vi "excavator1D_singleSet.vi"(4 "x Max":dbl format="%#_13g", 6 "x Min":dbl format="%#_13g", 9 "Limits":bool=TRUE, 10 "Index Selection":dbl[](graph)=[-5.5039248036337095e-05, 0.002307601651409641, 0.0019375252973986789, 0.0020539827004540713, 0.0018766465480439364, 0.002005471562733874, 0.0019512440951075405, 0.0019016214297153055, 0.0020314427267294375, 0.0021225218602921813, 0.0020813973096664995, 0.0022190025250893087, 0.001999956712825224, 0.0021371180017013105, 0.0022027734317816793, 0.0022226846020203085, 0.0021817092376295475, 0.0022948075755266474, 0.0022634134918916972, 0.0024800556187983603, 0.0024709631223231556, 0.0024774496152531354, 0.0025178377341944723, 0.002528270776383579, 0.0024779048399068415, 0.0024436424602754412, 0.002515299420338124, 0.002657992171589285, 0.002703678625402972, 0.0027635940117761494, 0.0026640722469892355, 0.0028217502404004335, 0.002767086564563215, 0.0027189288404770194, 0.002773431036621332, 0.002864902134751901, 0.0028404979093465954, 0.0028498102794401346, 0.0029649439034983515, 0.002844457468017936, 0.0028746504918672144, 0.0026685349992476405, 0.002743897819891572, 0.0028248644433915616, 0.002763545874040574, 0.0026688438490964474, 0.0026700377056840807, 0.0024837456992827358, 0.002380804240237922, 0.0024809345486573875, 0.0024448799376841635, 0.002402537123998627, 0.0024637061171233652, 0.0022932857275009154, 0.002131347142858431, 0.0022557196440175175, 0.0021800588699989023, 0.0021162735123652966, 0.0020641911192797124, 0.00210531207267195, 0.0022086400946136563, 0.001933887047925964, 0.002116878272499889, 0.0022065737983211872, 0.0020789780362974854, 0.0020607836777344346, 0.002077205339446664, 0.0021651801478583367, 0.0022058752714656294, 0.0022308619110845028, 0.002125738380709663, 0.0022845100960694254, 0.0021997722215019166, 0.0022234479489270597, 0.002461879176553339, 0.0025202257151249797, 0.0027610767225269227, 0.0025679582846350967, 0.0027760936878621577, 0.0029153746319934724, 0.002828183607198298, 0.002911771065555513, 0.002850099717034027, 0.003011852188501507, 0.002978001633891836, 0.0030534794554114343, 0.0032127083861269055, 0.003229459561407566, 0.0032388945226557555, 0.0032649051398038866, 0.0034539019456133247, 0.003314487461466342, 0.003523444349411875, 0.0032591138617135583, 0.003294491511769593, 0.003397454728838056, 0.0034086612984538076, 0.003363308252301067, 0.0035417634062469006, 0.0033399937790818514, 0.0034248353447765114, 0.003367754106875509, 0.0033597103436477484, 0.0033762263017706575, 0.0032008031965233387, 0.0032906924025155604, 0.003052685607690364, 0.003188005741685629, 0.0031751723494380713, 0.0031929326243698595, 0.0030400021001696586, 0.0028970208135433496, 0.0029620371758937837, 0.002946394798345864, 0.0028604958381038157, 0.002807711868081242, 0.0028404531418345868, 0.002868238207884133, 0.002771933143958449, 0.0028260866762138902, 0.0028528206632472573, 0.0028678092872723936, 0.0027899347536731512, 0.002760024246526882, 0.002831580874044448, 0.0027767036808654666, 0.0027371311327442525, 0.002827920182608068, 0.0030329054221510886, 0.0031421066960319877, 0.0031102296547032894, 0.0030996970483101903, 0.003247960680164397, 0.0028167950338684024, 0.0030843265587463973, 0.003308130835648626, 0.0033440372557379306, 0.003310535824857652, 0.003259662224445492, 0.003445134102366865, 0.0036248990218155086, 0.003514034498948604, 0.003342654788866639, 0.003707280964590609, 0.003718612529337406, 0.0036582897300831974, 0.0037778353202156723, 0.0036167260841466486, 0.00371461093891412, 0.0037952737184241414, 0.0039342561503872275, 0.003733250347431749, 0.0036644286708906295, 0.003758999495767057, 0.003727773274295032, 0.003952888981439173, 0.003977277246303856, 0.0037454716744832694, 0.0040516692213714125, 0.004073583579156548, 0.004025802714750171, 0.004011987871490419, 0.0039272750378586355, 0.003968243941199034, 0.004197335022035986, 0.0040430625551380215, 0.0037808504421263933, 0.004111979086883366, 0.0038525969488546253, 0.004002017085440457, 0.003939462278503924, 0.004101991350762546, 0.004090622591320425, 0.004113064985722304, 0.004230326088145375, 0.0038941988837905227, 0.004035194672178477, 0.004230266809463501, 0.004063357424456626, 0.003882370889186859, 0.004050530272070319, 0.004262716963421553, 0.004161569278221577, 0.004185240180231631, 0.004006734420545399, 0.004328481166157872, 0.004279951227363199, 0.004003130178898573, 0.004054784483741969, 0.00410827990854159, 0.0041830478352494534, 0.003808241744991392, 0.004008986777625978, 0.004141540615819395, 0.004094414797145873, 0.0040222823270596566, 0.003910915646702051, 0.0038658810313791036, 0.0038650343543849886, 0.0037868338637053966, 0.004014773108065128, 0.0038762923213653266, 0.003976433048956096, 0.003925886924844235, 0.003934970719274134, 0.0040465979371219875, 0.003861211775802076, 0.0038268946111202243, 0.003694956109393388, 0.003924443002324552, 0.0037448840332217513, 0.003946416464168578, 0.003847979276906699, 0.0038791699684225024, 0.00395004382589832, 0.004012362146750092, 0.003845076134894043, 0.0037047052290290596, 0.003880892100278288, 0.003927376854699105, 0.003974233590997756, 0.0042317162966355685, 0.004147131089121103, 0.004217348399106413, 0.004303383931983262, 0.004251424223184586, 0.004328834661282599, 0.004337806510739029, 0.00430601512780413, 0.004701763018965721, 0.004609443340450525, 0.004648852930404246, 0.00466197885107249, 0.004469169932417571, 0.004529011272825301, 0.004784878226928413, 0.0047280876198783515, 0.004763454629573971, 0.004759062337689101, 0.004903659271076321, 0.004659748158883303, 0.004927646089345217, 0.00475729265017435, 0.004669046879280358, 0.0047808624105527995, 0.0048078475869260725, 0.004636365990154445, 0.0048046133946627375, 0.00481757263187319, 0.004802378546446562, 0.004693611955735833, 0.004651836957782507, 0.004759728745557368, 0.004840704170055688, 0.004631528840400278, 0.00448742148000747, 0.004653911094646901, 0.00436076499754563, 0.004473710199818015, 0.004461665241979063, 0.004512202413752675, 0.004511458578053862, 0.0045105037046596404, 0.0044299363042227926, 0.004531701223459095, 0.004217351053375751, 0.004368505894672125, 0.004261411097832024, 0.0044176482711918656, 0.004463766061235219, 0.004451539262663573, 0.004323075187858194, 0.00432194754248485, 0.004393766552675515, 0.0042924596345983446, 0.004546674247831106, 0.004421514715068042, 0.004494644771330059, 0.004661913902964443, 0.004492968961130828, 0.004474510159343481, 0.004593179386574775, 0.004743144928943365, 0.004724432772491127, 0.0047914121532812715, 0.004951085732318461, 0.004936700244434178, 0.005089287087321281, 0.0050569199025630954, 0.005180290504358709, 0.005009520438034087, 0.005052786623127759, 0.005131706641986966, 0.005228332336992025, 0.005075493454933166, 0.005141002452000975, 0.005470275576226413, 0.005277567519806325, 0.0052113591227680445, 0.005557392607443035, 0.00528640653938055, 0.0055864242836833, 0.0052565854974091055, 0.005369229684583842, 0.005361709976568818, 0.005379944620653987, 0.005324042169377208, 0.005494691431522369, 0.005203793710097671, 0.005568335112184286, 0.005295956926420331, 0.005314707965590059, 0.005401723389513791, 0.0054991618031635875, 0.005587166151963175, 0.005336340819485486, 0.005255989544093609, 0.005496206833049655, 0.0054799888748675585, 0.0054559961427003145, 0.005375558976083994, 0.00516069121658802, 0.005235537793487311, 0.005287682497873902, 0.005408188770525157, 0.0052254452835768465, 0.005474191741086543, 0.005263954238034784, 0.0055487087927758695, 0.005501159047707915, 0.005381059693172574, 0.005320573598146439, 0.005287946970202029, 0.005535849020816386, 0.005299185402691364, 0.005417378270067275, 0.005279678734950721, 0.005510361935012043, 0.005502240709029138, 0.005368484533391893, 0.005572396842762828, 0.0054582339245826, 0.005252901371568442, 0.005599887482821942, 0.005541052296757698, 0.005322722741402686, 0.005597052932716906, 0.0053835853701457385, 0.00543387858197093, 0.0057798660127446055, 0.005603539990261197, 0.0053190829697996374, 0.00555386368650943, 0.005498887016437947, 0.00568358525633812, 0.005729269608855248, 0.005587581847794354, 0.005761724547483027, 0.005647446285001934, 0.005777251394465566, 0.005751495040021837, 0.005840469431132078, 0.005701329186558723, 0.005910418857820332, 0.005600121850147843, 0.005697100632824003, 0.0058915694011375305, 0.005879594711586833, 0.0058825223473832015, 0.005831844871863723, 0.005880430480465293, 0.005932610156014561, 0.005944398534484208, 0.005719918943941593, 0.005835889000445605, 0.005884684156626463, 0.00584760659839958, 0.0058321917429566385, 0.005720162182115018, 0.005849101720377803, 0.0058104357914999126, 0.005852596717886627, 0.006050111562944949, 0.006002284912392497, 0.005917288758791983, 0.0056698916014283895, 0.005833093030378223, 0.005962672969326377, 0.0059752183267846705, 0.005824555293656886, 0.005792977754026651, 0.006099943607114256, 0.0060348108410835264, 0.005918262735940516, 0.006149726593866944, 0.005918244109489023, 0.005964341573417187, 0.006059793778695166, 0.00594170477706939, 0.005921040661633015, 0.005834951857104897, 0.005985226575285196, 0.005786735098809004, 0.006013568490743637, 0.005970848142169416, 0.006068194750696421, 0.0058811110444366935, 0.0061480032047256826, 0.005966368853114546, 0.006032922049053013, 0.005986752943135798, 0.005800247448496521, 0.006086162896826864, 0.00608808824326843, 0.006292875786311924, 0.005918822344392538, 0.006007107626646757, 0.006163849052973092, 0.005986041901633143, 0.006119643454439938, 0.006091755745001137, 0.006163161643780768, 0.006068358686752618, 0.006234377133660018, 0.006458197068423033, 0.006379976100288331, 0.0063821553951129316, 0.006177129549905657, 0.006110375537537039, 0.006422333535738289, 0.0064666233723983165, 0.006352819106541574, 0.006392215238884091, 0.006317960936576128, 0.006309068389236927, 0.0063511111540719865, 0.006384995835833252, 0.0064990100450813765, 0.0064924719976261255, 0.006661783996969461, 0.006618827674537897, 0.006453927676193416, 0.006605154578574002, 0.006483975914306939, 0.006546729966066778, 0.006742855487391353, 0.006628313637338579, 0.006576768145896495, 0.006522198393940926, 0.00667329381685704, 0.006488177296705544, 0.0066192809259518984, 0.006664956011809409, 0.00666686212643981, 0.006601663213223219, 0.006686174753122031, 0.006772608147002757, 0.006783138355240226, 0.006614528829231858, 0.006824186886660755, 0.0064020713325589895, 0.00666458704508841, 0.006660054204985499, 0.0066425914876163, 0.00685013581532985, 0.00680395367089659, 0.0069337900262326, 0.006734993145801127, 0.00682165608741343, 0.006791043351404369, 0.006903514172881842, 0.006652213563211262, 0.006880231574177742, 0.006973042385652661, 0.006618744600564242, 0.006916143582202494, 0.006781034357845783, 0.006806752714328468, 0.007038682233542204, 0.006947669666260481, 0.0070041322614997625, 0.006932605500333012, 0.00701547390781343, 0.00697906028944999, 0.007335847592912614, 0.007086012186482549, 0.007146704779006541, 0.007008162187412382, 0.007009716215543449, 0.007137610204517841, 0.006982554541900754, 0.007046666392125189, 0.006997882155701518, 0.007004353683441877, 0.007141475402750075, 0.007233784161508083, 0.007191896950826049, 0.007311815279535949, 0.007185101229697466, 0.007161983009427786, 0.007202247041277587]) -> ()   [LabVIEW 2013]
panel:
  in  "Tab Control":enum32{"Page 1", "Page 2"}(tab)
  in  "All data or only selected?":bool
  out "xPoints":i32=263
  in  "Save File":path
  # "All Data"
  # "Data on graph"
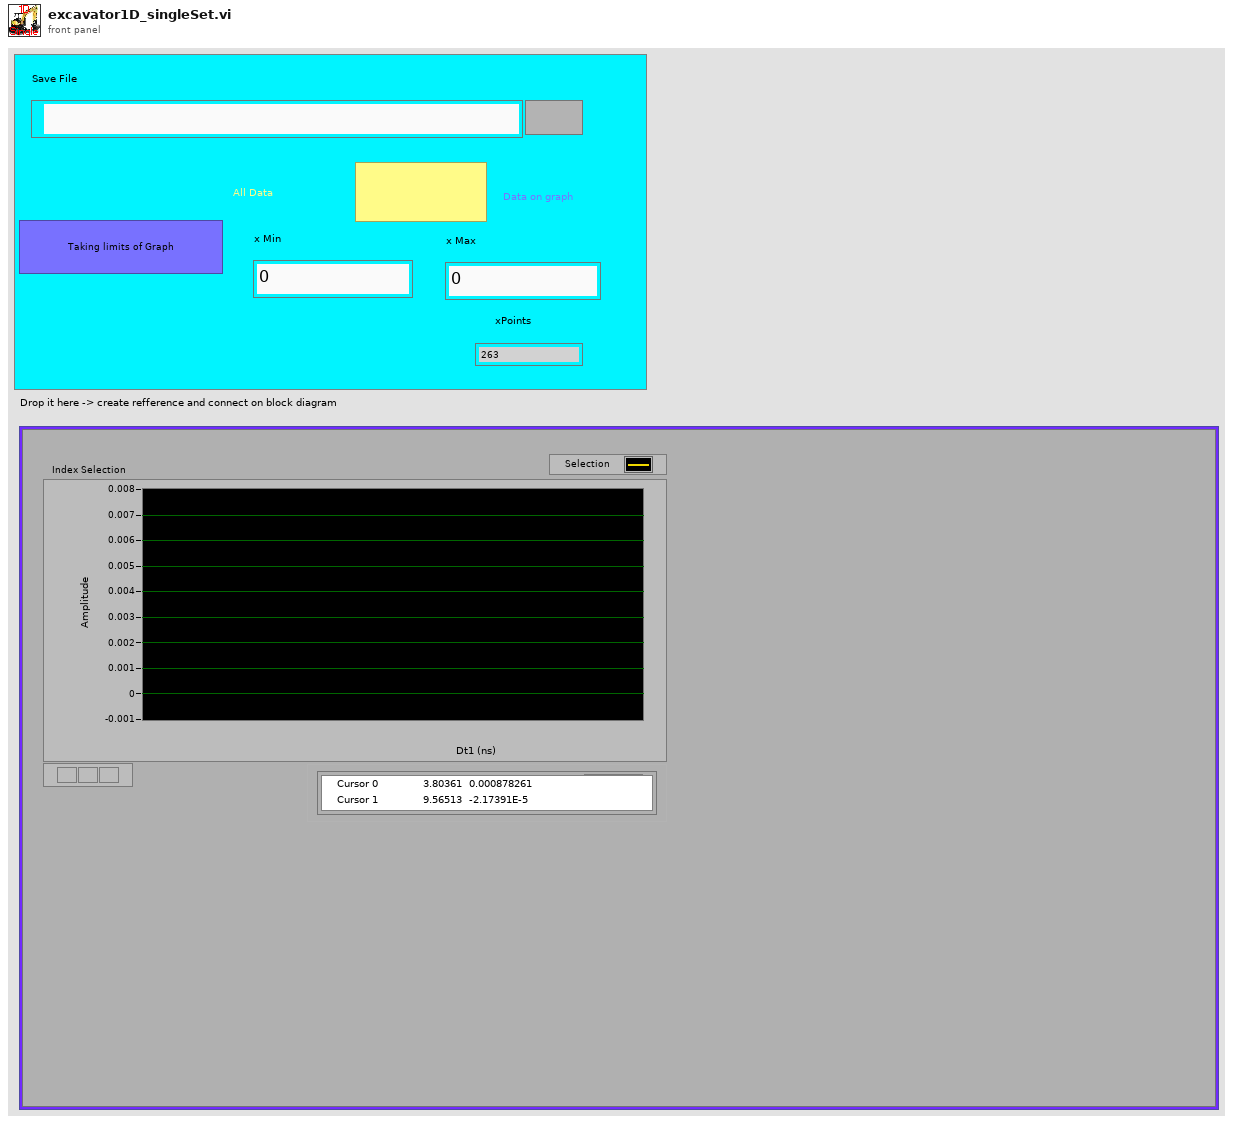
[diagram p1: front panel]
types:
  T1 = enum16{"open", "replace", "create", "open or create", "replace or create", "replace or create with confirmation"}
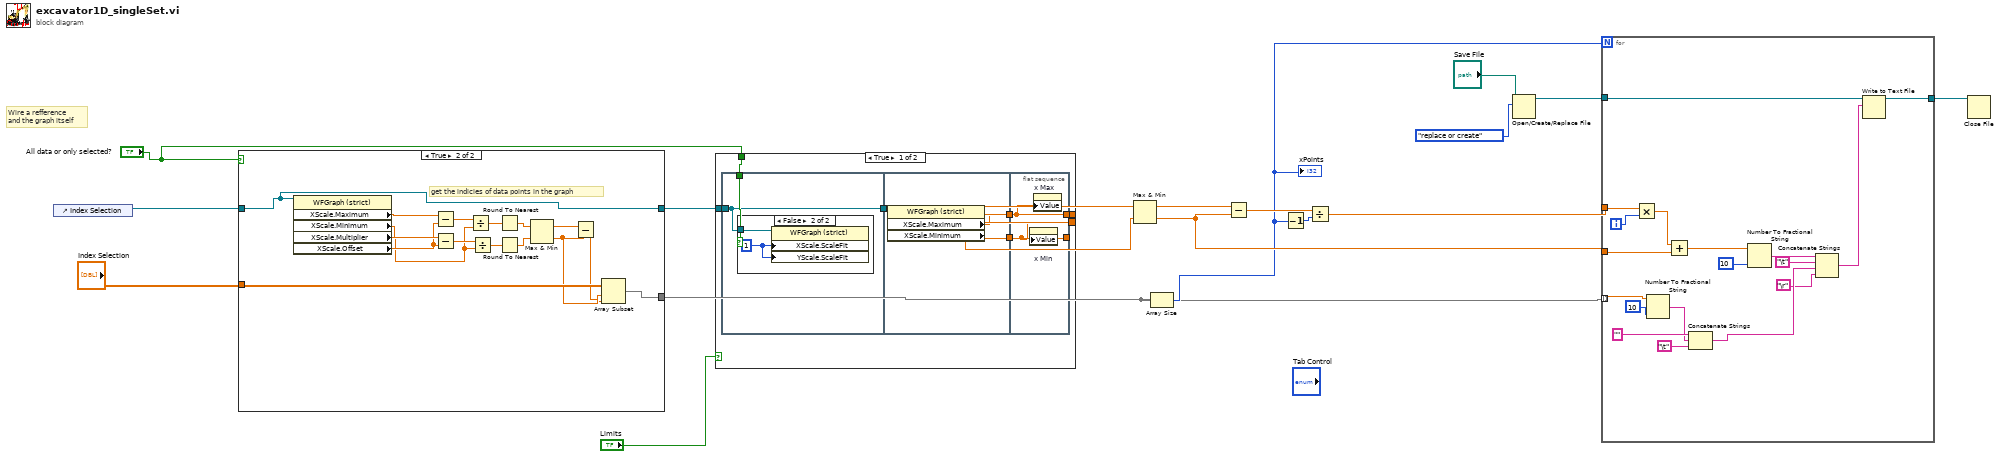
[diagram p0: block diagram]
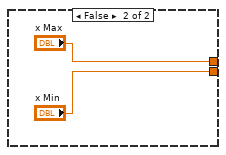
[diagram p4: hidden frame]
diagram:
  # "Wire a refference\nand the graph itself"
  n1 = control-ref of="Index Selection"() -> (w3:refnum<vi>)
  n2 = case shown="True" "All data or only selected?" {
    tunnel: "Index Selection" -> [w20 w25]
    tunnel: w3 -> [w19 w23]
    tunnel: [w20 w24] -> w4
    tunnel: [w19 w23] -> w12
    frame False {
    }
    frame True {
      # "get the indicies of data points in the graph"
      n3 = property class="WFGraph (strict)"(reference=w23) -> ("XScale.Maximum"=w33:dbl, "XScale.Minimum"=w36:dbl, "XScale.Multiplier"=w29:dbl, "XScale.Offset"=w30:dbl)  [unwired: 1 in, 2 out]
      n4 = Subtract(x=w33, y=w30) -> (x-y=w34:dbl)
      n5 = Subtract(x=w36, y=w30) -> (x-y=w35:dbl)
      n6 = Divide(x=w34, y=w29) -> (x/y=w32:dbl)
      n7 = Divide(x=w35, y=w29) -> (x/y=w31:dbl)
      n8 = Round To Nearest(number=w32) -> (nearest integer value=w28:dbl)
      n9 = Round To Nearest(number=w31) -> (nearest integer value=w27:dbl)
      n10 = Max & Min(x=w28, y=w27) -> (max(x,y)=w26:dbl, min(x,y)=w22:dbl)
      n11 = Subtract(x=w26, y=w22) -> (x-y=w21:dbl)
      n12 = Array Subset(array=w25, index=w22, length=w21) -> (w24:dbl[])
    }
  }
  n13 = case shown="True" "Limits" {
    tunnel: [w42 "x Max"] -> w10
    tunnel: [w41 "x Min"] -> w9
    tunnel: w12 -> [w43 _]
    tunnel: "All data or only selected?" -> [w39 _]
    frame True {
      n14 = flat-sequence {
        tunnel: w43 -> [w44]
        tunnel: [w44] -> w40
        tunnel: w39 -> [w45]
        tunnel: w40 -> [w50]
        tunnel: [w49] -> w38
        tunnel: [w48] -> w37
        tunnel: [w51] -> w41
        tunnel: [w52] -> w42
        tunnel: w38 -> [w52]
        tunnel: w37 -> [w51]
        frame #0 {
          n15 = case shown="False" w45 {
            tunnel: w44 -> [_ w46]
            frame True {
            }
            frame False {
              w47 = u8 1 ("X Scale.Scale Fit")
              n16 = property class="WFGraph (strict)"(reference=w46, "XScale.ScaleFit"=w47, "YScale.ScaleFit"=w47) -> ()  [unwired: 1 in, 2 out]
            }
          }
        }
        frame #1 {
          n17 = property class="WFGraph (strict)"(reference=w50) -> ("XScale.Maximum"=w49:dbl, "XScale.Minimum"=w48:dbl)  [unwired: 1 in, 2 out]
        }
        frame #2 {
          n18 = property on="x Min" class="DigNum (strict)"("Value"=w51) -> ()  [unwired: 2 in, 2 out]
          n19 = property on="x Max" class="DigNum (strict)"("Value"=w52) -> ()  [unwired: 2 in, 2 out]
        }
      }
    }
    frame False {
    }
  }
  n20 = Max & Min(x=w10, y=w9) -> (max(x,y)=w8:dbl, min(x,y)=w7:dbl)
  n21 = Array Size(array=w4) -> (size(s)=w5:i32)
  "xPoints" <- w5
  n22 = Subtract(x=w8, y=w7) -> (x-y=w14:dbl)
  n23 = Decrement(x=w5) -> (x-1=w6:i32)
  n24 = Divide(x=w14, y=w6) -> (x/y=w16:dbl)
  n25 = Open/Create/Replace File(file path (use dialog)="Save File", operation (0:open)=T1."replace or create") -> (refnum out=w18:refnum<file>)  [unwired: 4 in, 2 out]
  n26 = for {
    N: w5 -> [_]
    tunnel: w18 -> [w72]
    tunnel: w16 -> [w71]
    tunnel: w7 -> [w68]
    tunnel: [w66] -> w15
    tunnel: w4 -> [w55] mode=indexing
    i -> [w70]
    n27 = Multiply(x=w71, y=w70) -> (x*y=w69:dbl)
    n28 = Number To Fractional String(number=w55, precision (6)=i16 10 ("width (-)")) -> (F-format string=w58:string)  [unwired: 2 in]
    n29 = Add(x=w69, y=w68) -> (x+y=w67:dbl)
    n30 = Concatenate Strings("" ("string"), w58, "\t") -> (w60:string)
    n31 = Number To Fractional String(number=w67, precision (6)=i16 10 ("width (-)")) -> (F-format string=w65:string)  [unwired: 2 in]
    n32 = Concatenate Strings(w65, "\t", w60, "\r") -> (w64:string)
    n33 = Write to Text File(file (use dialog)=w72, text=w64) -> (refnum out=w66:refnum<file>)  [unwired: 2 in, 2 out]
  }
  n34 = Close File(refnum=w15) -> ()  [unwired: 1 in, 2 out]
